vi "DAQinit.vi"(2 "Tree Path In":string, 3 "error in (no error)":errorcluster, 4 "Digitizer Settings":T1, 5 "Data Value Reference in":refnum<data-value>) -> (0 "error out":errorcluster)   [LabVIEW 2013]
uses:
  <vilib>/MDSplus/Classes/Tree_Class/Tree.lvclass
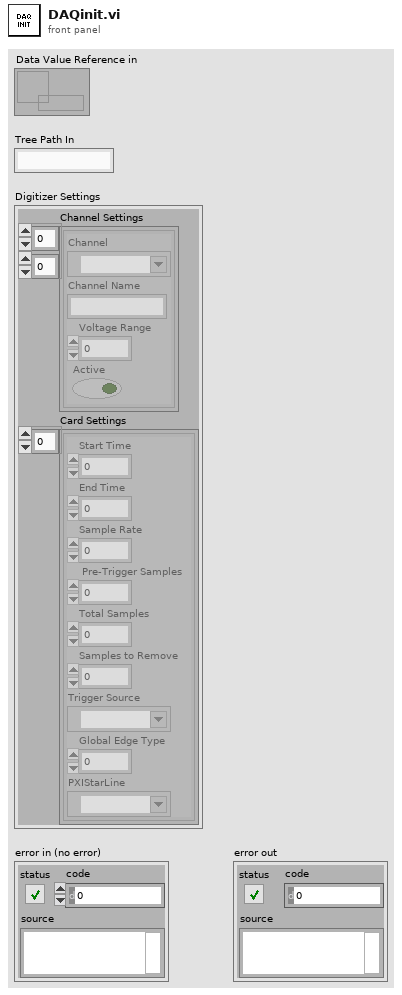
[diagram p1: front panel]
types:
  T1 = cluster{"Channel Settings":cluster{"Channel":tag, "Channel Name":string, "Voltage Range":dbl, "Active":bool}[][], "Card Settings":cluster{"Start Time":dbl, "End Time":dbl, "Sample Rate":dbl, " Pre-Trigger Samples":u32, "Total Samples":i32, "Samples to Remove":u32, "Trigger Source":tag, "Global Edge Type":i32, "PXIStarLine":tag}[]}
  T2 = cluster{"Channel":tag, "Channel Name":string, "Voltage Range":dbl, "Active":bool}[][]
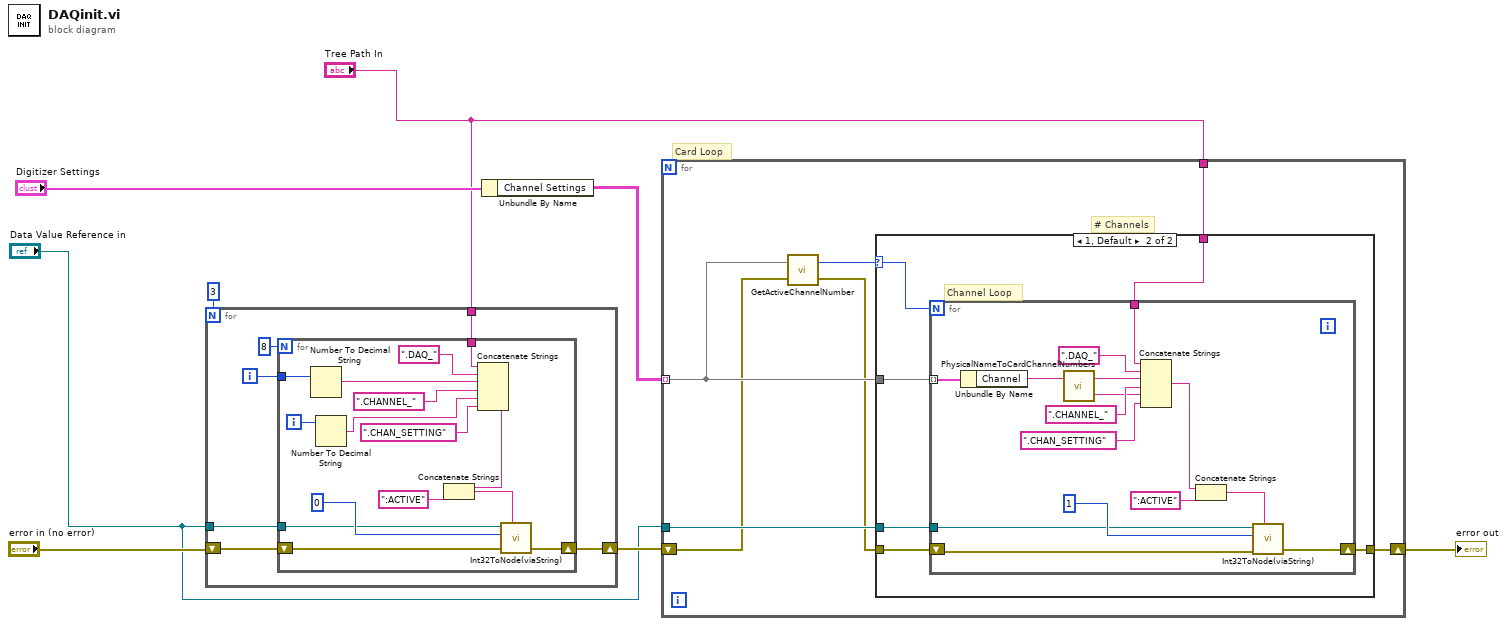
[diagram p0: block diagram]
diagram:
  # "Card Loop"
  n1 = for {
    N: 3 -> [_]
    shift-right: [w11] -> w4
    shift-left: "error in (no error)" -> [w12]
    tunnel: "Data Value Reference in" -> [w10]
    tunnel: "Tree Path In" -> [w9]
    i -> [w13]
    n2 = for {
      N: 8 -> [_]
      tunnel: w13 -> [w25]
      shift-right: [w15] -> w11
      shift-left: w12 -> [w16]
      tunnel: w10 -> [w18]
      tunnel: w9 -> [w17]
      i -> [w24]
      n3 = Number To Decimal String(number=w25) -> (decimal integer string=w26:string)  [unwired: 1 in]
      n4 = Number To Decimal String(number=w24) -> (decimal integer string=w23:string)  [unwired: 1 in]
      n5 = Concatenate Strings(w17, ".DAQ_" ("string"), w26, ".CHANNEL_" ("string"), w23, ".CHAN_SETTING" ("string")) -> (w20:string)
      n6 = Concatenate Strings(w20, ":ACTIVE" ("string")) -> (w22:string)
      n7 = call "Int32ToNode(viaString).vi"("Tree DVR in"=w18, "I32 in"=0, "error in (no error)"=w16, "NodePath"=w22) -> ("error out"=w15:errorcluster)  [unwired: 1 in, 2 out]
    }
  }
  n8 = Unbundle By Name("Digitizer Settings") -> ("Channel Settings"=w8:T2)
  n9 = for {
    tunnel: w8 -> [w36] mode=indexing
    tunnel: "Data Value Reference in" -> [w35]
    tunnel: "Tree Path In" -> [w34]
    shift-right: [w32] -> w1
    shift-left: w4 -> [w31]
    # "# Channels"
    n10 = call "GetActiveChannelNumber.vi"("error in (no error)"=w31, "Channel Settings"=w36) -> ("error out"=w33:errorcluster, "Numeric"=w30:i32)
    n11 = case shown="1, Default" w30 {
      selector: w30 -> [_ w38]
      tunnel: w36 -> [_ w43]
      tunnel: w35 -> [_ w42]
      tunnel: w34 -> [_ w41]
      tunnel: w33 -> [w37 w40]
      tunnel: [w37 w39] -> w32
      frame 0 {
      }
      frame 1, Default {
        # "Channel Loop"
        n12 = for {
          N: w38 -> [_]
          tunnel: w41 -> [w52]
          tunnel: w43 -> [w51] mode=indexing
          tunnel: w42 -> [w46]
          shift-right: [w45] -> w39
          shift-left: w40 -> [w47]
          n13 = Unbundle By Name(w51) -> ("Channel"=w54:tag)
          n14 = call "PhysicalNameToCardChannelNumbers.vi"("NI Physical Channel"=w54) -> ("Channel #"=w55:string, "Card #"=w56:string)  [unwired: 1 in]
          n15 = Concatenate Strings(w52, ".DAQ_" ("string"), w56, ".CHANNEL_" ("string"), w55, ".CHAN_SETTING" ("string")) -> (w44:string)
          n16 = Concatenate Strings(w44, ":ACTIVE" ("string")) -> (w50:string)
          n17 = call "Int32ToNode(viaString).vi"("Tree DVR in"=w46, "I32 in"=1, "error in (no error)"=w47, "NodePath"=w50) -> ("error out"=w45:errorcluster)  [unwired: 1 in, 2 out]
        }
      }
    }
  }
  "error out" <- w1
